vi "configure build specification.vi"(6 "pre and post build refs":refnum<vi>[](array[refnum]), 7 "plugin name":string, 8 "error in (no error)":errorcluster, 9 "version information":T1, 10 "root folder path":path, 11 "Project ref in":refnum<vi>) -> (0 "error out":errorcluster, 3 "NI_AB_API_PPL out":refnum<class "NI_AB_API_PPL.lvclass">)   [LabVIEW 2024]
doc: "configures and creates a packed library build specification within the target lvproj file"
uses:
  <vilib>/AppBuilder/AB_API/PPL/NI_AB_API_PPL.lvclass
  <vilib>/AppBuilder/AB_API/common/AB_API Version Information.ctl
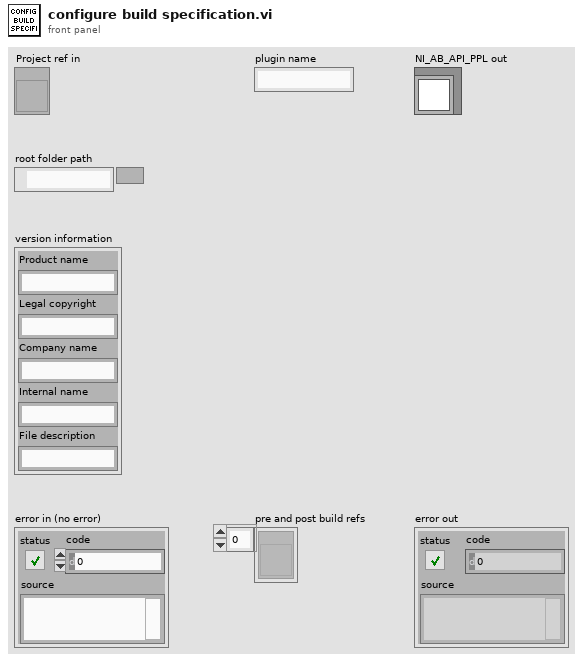
[diagram p1: front panel]
types:
  T1 = typedef "AB_API Version Information.ctl" = cluster{"Product name":string, "Legal copyright":string, "Company name":string, "Internal name":string, "File description":string}
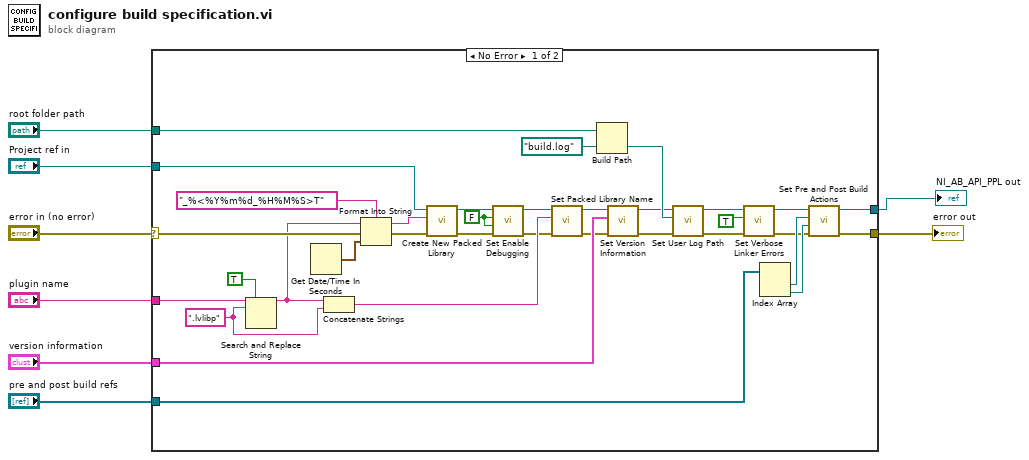
[diagram p0: block diagram]
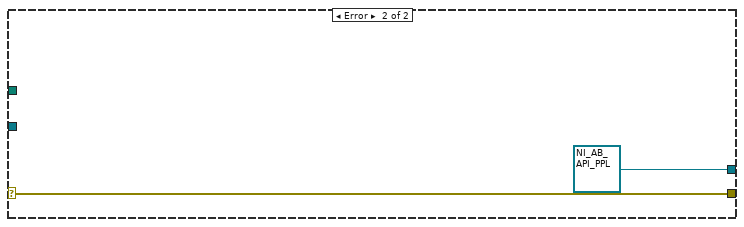
[diagram p2: hidden frame]
diagram:
  n1 = case shown="No Error" "error in (no error)" {
    selector: "error in (no error)" -> [w42 w44]
    tunnel: "Project ref in" -> [w41 _]
    tunnel: "pre and post build refs" -> [w40 _]
    tunnel: "plugin name" -> [w31 _]
    tunnel: "root folder path" -> [w26 _]
    tunnel: "version information" -> [w21 _]
    tunnel: [w13 refnum<class "NI_AB_API_PPL.lvclass"> refnum ("Build out")] -> w2
    tunnel: [w11 w44] -> w1
    frame No Error {
      w38 = ".lvlibp" ("search string")
      w17 = FALSE ("Enable debugging (false)")
      n2 = Search and Replace String(replace all?=TRUE ("replace all? (F)"), input string=w31, search string=w38) -> (result string=w36:string)  [unwired: 5 in, 3 out]
      n3 = Get Date/Time In Seconds() -> (seconds since 1Jan1904=w33:timestamp)
      n4 = Concatenate Strings(w36, w38) -> (w37:string)
      n5 = Format Into String(format string="_%<%Y%m%d_%H%M%S>T", initial string=w36, error in=w42, w33) -> (resulting string=w34:string, error out=w35:errorcluster)
      n6 = call <vilib>:"Create New Packed Library.vi"("error in (no error)"=w35, "Build specification name"=w34, "Project Refnum"=w41) -> ("error out"=w14:errorcluster, "PPL out"=w16:refnum<class "NI_AB_API_PPL.lvclass">)  [unwired: 7 in]
      n7 = call-dynamic "Set Enable Debugging.vi"("error in (no error)"=w14, "Wait for debugger on launch (false)"=w17, "Enable debugging (false)"=w17, "PPL in"=w16) -> ("error out"=w15:errorcluster, "PPL out"=w18:refnum<class "NI_AB_API_PPL.lvclass">)  [unwired: 6 in]
      n8 = call-dynamic "Set Packed Library Name.vi"("error in (no error)"=w15, "Packed library name"=w37, "PPL in"=w18) -> ("error out"=w20:errorcluster, "PPL out"=w19:refnum<class "NI_AB_API_PPL.lvclass">)  [unwired: 7 in]
      n9 = Build Path(base path=w26, name or relative path=path "build.log") -> (appended path=w27:path)
      n10 = call-dynamic "Set Version Information.vi"("error in (no error)"=w20, "Version Information"=w21, "PPL in"=w19) -> ("error out"=w23:errorcluster, "PPL out"=w22:refnum<class "NI_AB_API_PPL.lvclass">)  [unwired: 7 in]
      n11 = call-dynamic "Set User Log Path.vi"("error in (no error)"=w23, "user log path"=w27, "NI_AB_API_PPL in"=w22) -> ("error out"=w24:errorcluster, "NI_AB_API_PPL out"=w25:refnum<class "NI_AB_API_PPL.lvclass">)  [unwired: 7 in]
      n12 = call-dynamic "Set Verbose Linker Errors.vi"("error in (no error)"=w24, "Verbose Linker Errors? (true)"=TRUE, "PPL in"=w25) -> ("error out"=w10:errorcluster, "PPL out"=w12:refnum<class "NI_AB_API_PPL.lvclass">)  [unwired: 7 in]
      n13 = Index Array(array=w40) -> (element #1=w29:refnum<vi>, element #2=w30:refnum<vi>)  [unwired: 2 in]
      n14 = call-dynamic "Set Pre and Post Build Actions.vi"("error in (no error)"=w10, "Post Build Action VI"=w30, "Pre Build Action VI"=w29, "Build in"=w12) -> ("error out"=w11:errorcluster, "Build out"=w13:refnum<class "NI_AB_API_PPL.lvclass">)  [unwired: 6 in]
    }
    frame Error {
    }
  }
  "NI_AB_API_PPL out" <- w2
  "error out" <- w1
